vi "SigGen-Compute Max Level (full wrapper).vi"(0 "Stimulus Channel":T1={"Waveform"={"Type"=enum."OFF", "Tone"={"Frequency (kHz)"=0.0, "Last Freq"=0.0, "Last Phase"=0.0}, "Pulse Train"={"Pulse width (us)"=0.0, "Pulse rate (Hz)"=0.0, "Gap (ms)"=0.0, "Polarity"=enum."POS", "PT State"={"Template"=[], "Nperiod"=0, "Index"=0, "Pulse Rate (Hz)"=0.0, "Phase (cycles)"=0.0, "Noff"=0}, "Asynch"=FALSE}, "Noise"={"InvFilt"=FALSE, "Noise"=[], "CurPt"=0, "Aweight"=FALSE, "Seed"=0, "afile"=path ""}, "File"={"Filename"=path "", "Signal"=[], "Channel"=0, "stream"=FALSE, "offset"=0, "nreps"=0, "loops"=0, "Randomize"=FALSE, "order"=[], "Seed"=0, "Tokens"=0}, "FMSweep"={"Rate (oct/s)"=0.0, "Fmin (Hz)"=0.0, "Fmax (Hz)"=0.0, "Ramp (ms)"=0.0, "Linear"=FALSE}, "Chirp Train"={"Params"={"Fmin (kHz)"=4.0, "Fmax (kHz)"=64.0, "Compensate"=FALSE, "Duration (ms)"=2.0}, "Data"={"WF"=[]}}, "Complex Tone"={"Params"={"F0 (Hz)"=0.0, "Band"={"Flow (Hz)"=0.0, "Fhigh (Hz)"=0.0}, "Phase"=enum."Cosine", "Min F0 (Hz)"=0.0, "Max F0 (Hz)"=0.0, "ContinRandPhase"=FALSE, "Max peak factor"=inf, "Max mod depth"=2.0, "MinHarmNum"=0, "MaxHarmNum"=0, "Level Mode"=enum."per component", "% jitter"=0.0}, "Data"={"Ncomp"=0, "MinHarm"=0, "Phase"=[], "Amplitude"=[], "Npts/frame"=0, "Last F0"=0.0, "Fmin"=0.0, "Fmax"=0.0, "Lslope"=0.0, "randphase"=FALSE, "overall rms"=FALSE, "fmult"=[], "jittered"=FALSE}}, "Moving Ripple"={"Params"={"Fmin"=0.0, "Fmax"=0.0, "Density"=0.0, "Velocity"=0.0, "Depth"=0.0, "Phase"=0.0, "Comp/oct"=0}, "Data"={"Freq"=[], "A"=[], "phase"=[], "Phase"=0.0}}}, "Filter"={"Type"=enum."Lowpass", "CF (kHz)"=0.0, "BW (kHz)"=0.0, "Cascade"=FALSE, "Quadrature"=FALSE, "Scale Factor"=0.0, "Stages"=[], "Class"=enum."Elliptic", "Order"=0, "BWUnits"=enum."Linear"}, "Burst"={"Active"=FALSE, "Delay (ms)"=0.0, "Duration (ms)"=0.0, "Ramp (ms)"=0.0, "Rate (Hz)"=0.0, "Trepeat (ms)"=0.0, "Repeat"=FALSE}, "Level"={"Level"=0.0, "Units"=enum."dB atten", "Max"=0.0, "Multiplier"=0.0, "Cal File"=path "", "Cal"={"Freq (Hz)"=[], "Mag (dB SPL)"=[], "Phase (deg)"=[]}}, "Name"="", "Advanced"={"Rep Mask"="", "AltPol"=FALSE, "Var"="", "Expr"="", "Persist"=FALSE}, "SAM"={"Active"=FALSE, "Frequency (Hz)"=0.0, "Depth"=0.0, "Init Phase (cycles)"=0.0, "phase (degrees)"=0.0, "Asynch"=FALSE}} {"Filter"."Stages"."IIR Filter"."Forward Coefficients" format="%.4f"; "Filter"."Stages"."IIR Filter"."Reverse Coefficients" format="%.4f"}, 7 "Sampling Rate (Hz)":dbl, 9 "Npts":i32, 11 "error in (no error)":errorcluster) -> (4 "Stimulus Channel out":T1={"Waveform"={"Type"=enum."OFF", "Tone"={"Frequency (kHz)"=0.0, "Last Freq"=0.0, "Last Phase"=0.0}, "Pulse Train"={"Pulse width (us)"=0.0, "Pulse rate (Hz)"=0.0, "Gap (ms)"=0.0, "Polarity"=enum."POS", "PT State"={"Template"=[], "Nperiod"=0, "Index"=0, "Pulse Rate (Hz)"=0.0, "Phase (cycles)"=0.0, "Noff"=0}, "Asynch"=FALSE}, "Noise"={"InvFilt"=FALSE, "Noise"=[], "CurPt"=0, "Aweight"=FALSE, "Seed"=0, "afile"=path ""}, "File"={"Filename"=path "", "Signal"=[], "Channel"=0, "stream"=FALSE, "offset"=0, "nreps"=0, "loops"=0, "Randomize"=FALSE, "order"=[], "Seed"=0, "Tokens"=0}, "FMSweep"={"Rate (oct/s)"=0.0, "Fmin (Hz)"=0.0, "Fmax (Hz)"=0.0, "Ramp (ms)"=0.0, "Linear"=FALSE}, "Chirp Train"={"Params"={"Fmin (kHz)"=4.0, "Fmax (kHz)"=64.0, "Compensate"=FALSE, "Duration (ms)"=2.0}, "Data"={"WF"=[]}}, "Complex Tone"={"Params"={"F0 (Hz)"=0.0, "Band"={"Flow (Hz)"=0.0, "Fhigh (Hz)"=0.0}, "Phase"=enum."Cosine", "Min F0 (Hz)"=0.0, "Max F0 (Hz)"=0.0, "ContinRandPhase"=FALSE, "Max peak factor"=inf, "Max mod depth"=2.0, "MinHarmNum"=0, "MaxHarmNum"=0, "Level Mode"=enum."per component", "% jitter"=0.0}, "Data"={"Ncomp"=0, "MinHarm"=0, "Phase"=[], "Amplitude"=[], "Npts/frame"=0, "Last F0"=0.0, "Fmin"=0.0, "Fmax"=0.0, "Lslope"=0.0, "randphase"=FALSE, "overall rms"=FALSE, "fmult"=[], "jittered"=FALSE}}, "Moving Ripple"={"Params"={"Fmin"=0.0, "Fmax"=0.0, "Density"=0.0, "Velocity"=0.0, "Depth"=0.0, "Phase"=0.0, "Comp/oct"=0}, "Data"={"Freq"=[], "A"=[], "phase"=[], "Phase"=0.0}}}, "Filter"={"Type"=enum."Lowpass", "CF (kHz)"=0.0, "BW (kHz)"=0.0, "Cascade"=FALSE, "Quadrature"=FALSE, "Scale Factor"=0.0, "Stages"=[], "Class"=enum."Elliptic", "Order"=0, "BWUnits"=enum."Linear"}, "Burst"={"Active"=FALSE, "Delay (ms)"=0.0, "Duration (ms)"=0.0, "Ramp (ms)"=0.0, "Rate (Hz)"=0.0, "Trepeat (ms)"=0.0, "Repeat"=FALSE}, "Level"={"Level"=0.0, "Units"=enum."dB atten", "Max"=0.0, "Multiplier"=0.0, "Cal File"=path "", "Cal"={"Freq (Hz)"=[], "Mag (dB SPL)"=[], "Phase (deg)"=[]}}, "Name"="", "Advanced"={"Rep Mask"="", "AltPol"=FALSE, "Var"="", "Expr"="", "Persist"=FALSE}, "SAM"={"Active"=FALSE, "Frequency (Hz)"=0.0, "Depth"=0.0, "Init Phase (cycles)"=0.0, "phase (degrees)"=0.0, "Asynch"=FALSE}} {"Filter"."Stages"."IIR Filter"."Forward Coefficients" format="%.4f"; "Filter"."Stages"."IIR Filter"."Reverse Coefficients" format="%.4f"}, 14 "Max Level":dbl, 15 "error out":errorcluster)   [LabVIEW 2020]
uses:
  Controls/Stimulus Channel (Full)/Full Stimulus Channel Data.ctl
  Controls/Waveform XCtl/Waveform Data.ctl
  Controls/Waveform XCtl/Waveform Enum.ctl
  Waveform VIs/Tone VIs/Tone Params.ctl
  Waveform VIs/Pulse Train VIs/Pulse Train Params.ctl
  Waveform VIs/Pulse Train VIs/Pulse Polarity.ctl
  Waveform VIs/Pulse Train VIs/PT-Continuous State.ctl
  Waveform VIs/Noise VIs/Noise Params.ctl
  Waveform VIs/File VIs/StimFile-Params.ctl
  Waveform VIs/FM Sweep VIs/FM Sweep Params.ctl
  Waveform VIs/Chirp Train VIs/Chirp Train.ctl
  Waveform VIs/Chirp Train VIs/Chirp Train Params.ctl
  Waveform VIs/Complex Tone VIs/CT-Params.ctl
  Waveform VIs/Complex Tone VIs/CT-Phase Enum.ctl
  Waveform VIs/Complex Tone VIs/CT-Runtime Data.ctl
  Waveform VIs/Moving Ripple VIs/Moving Ripple.ctl
  Waveform VIs/Moving Ripple VIs/Moving Ripple.Params.ctl
  Waveform VIs/Moving Ripple VIs/Moving Ripple.Data.ctl
  Controls/Advanced Filter XCtl/Filter Data.ctl
  Filter VIs/Filter-Bandwidth Units.ctl
  Controls/Burst XCtl/Burst Data.ctl
  Controls/Level XCtl/Level Data.ctl
  Controls/Level XCtl/Level Units.ctl
  Controls/Advanced Options XCtl/Advanced Stimulus Options.ctl
  Modulation VIs/SAM VIs/SAM Params.ctl
  Controls/Advanced Filter XCtl/Advanced Filter XCtl.xctl
  Controls/Level XCtl/Level XCtl.xctl
  Controls/Burst XCtl/Burst Control.xctl
  Controls/Waveform XCtl/Waveform XCtl.xctl
  Controls/Advanced Options XCtl/Advanced Stimulus Options.xctl
  Controls/Stimulus Channel (Full)/Stimulus Channel (Full).xctl
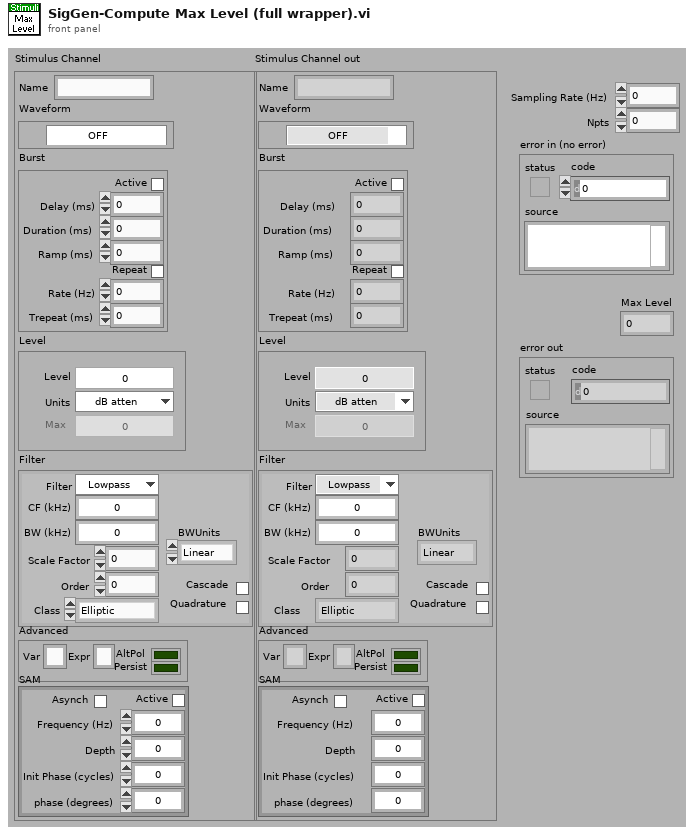
[diagram p1: front panel]
types:
  T1 = typedef "Stimulus Channel (Full).xctl/Full Stimulus Channel Data.ctl" = cluster{"Waveform":T2, "Filter":T19, "Burst":T21, "Level":T22, "Name":string, "Advanced":T24, "SAM":T25}
  T2 = typedef "Waveform XCtl.xctl/Waveform Data.ctl" = cluster{"Type":T3, "Tone":T4, "Pulse Train":T5, "Noise":T8, "File":T9, "FMSweep":T10, "Chirp Train":T11, "Complex Tone":cluster{"Params":T13, "Data":T15}, "Moving Ripple":T16}
  T3 = typedef "Waveform Enum.ctl" = enum16{"OFF", "Tone", "Noise", "Pulse Train", "File", "FM Sweep", "Chirp Train", "Complex Tone", "FM Tone", "Moving Ripple"}
  T4 = typedef "Tone Params.ctl" = cluster{"Frequency (kHz)":dbl, "Last Freq":dbl, "Last Phase":dbl}
  T5 = typedef "Pulse Train Params.ctl" = cluster{"Pulse width (us)":dbl, "Pulse rate (Hz)":dbl, "Gap (ms)":dbl, "Polarity":T6, "PT State":T7, "Asynch":bool}
  T6 = typedef "Pulse Polarity.ctl" = enum16{"POS", "NEG", "POS-NEG", "NEG-POS"}
  T7 = typedef "PT-Continuous State.ctl" = cluster{"Template":dbl[], "Nperiod":i32, "Index":i32, "Pulse Rate (Hz)":dbl, "Phase (cycles)":dbl, "Noff":i32}
  T8 = typedef "Noise Params.ctl" = cluster{"InvFilt":bool, "Noise":dbl[], "CurPt":i32, "Aweight":bool, "Seed":i32, "afile":path}
  T9 = typedef "StimFile-Params.ctl" = cluster{"Filename":path, "Signal":dbl[], "Channel":i32, "stream":bool, "offset":i32, "nreps":i32, "loops":i32, "Randomize":bool, "order":i32[], "Seed":i32, "Tokens":i32}
  T10 = typedef "FM Sweep Params.ctl" = cluster{"Rate (oct/s)":dbl, "Fmin (Hz)":dbl, "Fmax (Hz)":dbl, "Ramp (ms)":dbl, "Linear":bool}
  T11 = typedef "Chirp Train.ctl" = cluster{"Params":T12, "Data":cluster{"WF":dbl[]}}
  T12 = typedef "Chirp Train Params.ctl" = cluster{"Fmin (kHz)":dbl, "Fmax (kHz)":dbl, "Compensate":bool, "Duration (ms)":dbl}
  T13 = typedef "CT-Params.ctl" = cluster{"F0 (Hz)":dbl, "Band":cluster{"Flow (Hz)":dbl, "Fhigh (Hz)":dbl}, "Phase":T14, "Min F0 (Hz)":dbl, "Max F0 (Hz)":dbl, "ContinRandPhase":bool, "Max peak factor":dbl, "Max mod depth":dbl, "MinHarmNum":i32, "MaxHarmNum":i32, "Level Mode":enum16{"per component", "overall rms"}, "% jitter":dbl}
  T14 = typedef "CT-Phase Enum.ctl" = enum16{"Cosine", "Random", "Alternating"}
  T15 = typedef "CT-Runtime Data.ctl" = cluster{"Ncomp":i32, "MinHarm":i32, "Phase":dbl[], "Amplitude":dbl[], "Npts/frame":i32, "Last F0":dbl, "Fmin":dbl, "Fmax":dbl, "Lslope":dbl, "randphase":bool, "overall rms":bool, "fmult":dbl[], "jittered":bool}
  T16 = typedef "Moving Ripple.ctl" = cluster{"Params":T17, "Data":T18}
  T17 = typedef "Moving Ripple.Params.ctl" = cluster{"Fmin":dbl, "Fmax":dbl, "Density":dbl, "Velocity":dbl, "Depth":dbl, "Phase":dbl, "Comp/oct":i32}
  T18 = typedef "Moving Ripple.Data.ctl" = cluster{"Freq":dbl[], "A":dbl[], "phase":dbl[], "Phase":dbl}
  T19 = typedef "Advanced Filter XCtl.xctl/Filter Data.ctl" = cluster{"Type":enum16{"Lowpass", "Highpass", "Bandpass", "Bandstop", "OFF"}, "CF (kHz)":dbl, "BW (kHz)":dbl, "Cascade":bool, "Quadrature":bool, "Scale Factor":dbl, "Stages":cluster{"IIR Filter":cluster{"filter structure":enum32{"IIR 2nd Order", "IIR 4th Order"}, "Reverse Coefficients":dbl[], "Forward Coefficients":dbl[]}, "State":dbl[]}[], "Class":enum16{"Elliptic", "Butterworth"}, "Order":i32, "BWUnits":T20}
  T20 = typedef "Filter-Bandwidth Units.ctl" = enum16{"Linear", "Octaves", "Min-Max"}
  T21 = typedef "Burst Control.xctl/Burst Data.ctl" = cluster{"Active":bool, "Delay (ms)":dbl, "Duration (ms)":dbl, "Ramp (ms)":dbl, "Rate (Hz)":dbl, "Trepeat (ms)":dbl, "Repeat":bool}
  T22 = typedef "Level XCtl.xctl/Level Data.ctl" = cluster{"Level":dbl, "Units":T23, "Max":dbl, "Multiplier":dbl, "Cal File":path, "Cal":cluster{"Freq (Hz)":dbl[], "Mag (dB SPL)":dbl[], "Phase (deg)":dbl[]}}
  T23 = typedef "Level Units.ctl" = enum16{"dB atten", "dB SPL", "dB re 1 Vrms", "dB V/Hz½", "mW", "dB HL", "Volts", "dB mW"}
  T24 = typedef "Advanced Stimulus Options.xctl/Advanced Stimulus Options.ctl" = cluster{"Rep Mask":string, "AltPol":bool, "Var":string, "Expr":string, "Persist":bool}
  T25 = typedef "SAM Params.ctl" = cluster{"Active":bool, "Frequency (Hz)":dbl, "Depth":dbl, "Init Phase (cycles)":dbl, "phase (degrees)":dbl, "Asynch":bool}
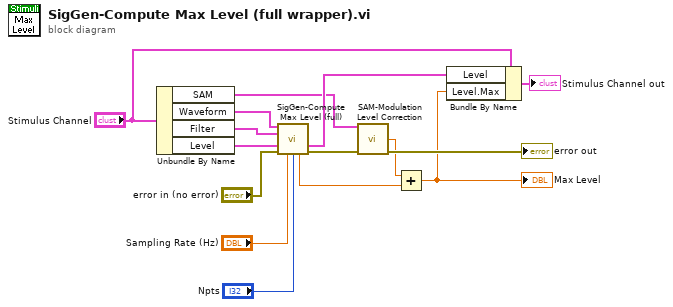
[diagram p0: block diagram]
diagram:
  n1 = Unbundle By Name("Stimulus Channel") -> ("SAM"=w3:T25, "Waveform"=w7:T2, "Filter"=w6:T19, "Level"=w15:T22)
  n2 = call "SigGen-Compute Max Level (full).vi"("Waveform"=w7, "Filter"=w6, "Level"=w15, "error in (no error)"="error in (no error)", "Sampling Rate (Hz)"="Sampling Rate (Hz)", "Npts"="Npts") -> ("Level out"=w9:T22, "Max Level"=w11:dbl, "error out"=w5:errorcluster)  [unwired: 7 in]
  n3 = call "SAM-Modulation Level Correction.vi"("SAM"=w3, "error in (no error)"=w5) -> ("Correction (dB)"=w2:dbl, "error out"=→"error out":errorcluster)  [unwired: 12 in]
  n4 = Add(x=w2, y=w11) -> (x+y=w1:dbl)
  "Max Level" <- w1
  n5 = Bundle By Name(cluster="Stimulus Channel", "Level"=w9, "Level.Max"=w1) -> (→"Stimulus Channel out":T1)
